vi "initialise.vi"(8 "error in (no error)":errorcluster, 11 "DL090211FrameImageAssembler in":refnum<class "ImageAssemblerDL090211Frame.lvclass">) -> (0 "error out":errorcluster, 3 "DL090211FrameImageAssembler out":refnum<class "ImageAssemblerDL090211Frame.lvclass">)   [LabVIEW 2010, in "ImageAssemblerDL090211Frame.lvclass"]
doc: "The dynamic dispatch-version of this VI initalises the plug-in object by allocating and initalising any dynamic resources need."
uses:
  ImageAssemblerDL090211Frame.lvclass
  ImageAssemblerDL090211Scaffold/ImageAssemblerDL090211Scaffold/ImageAssemblerDL090211Scaffold.lvclass
  common/arrays/pixel_raw_data_array.ctl
  ImageAssemblerDL090211Frame.lvclass/ImageAssemblerDL090211Frame.ctl
  common/classes/Image/Image/Image.lvclass
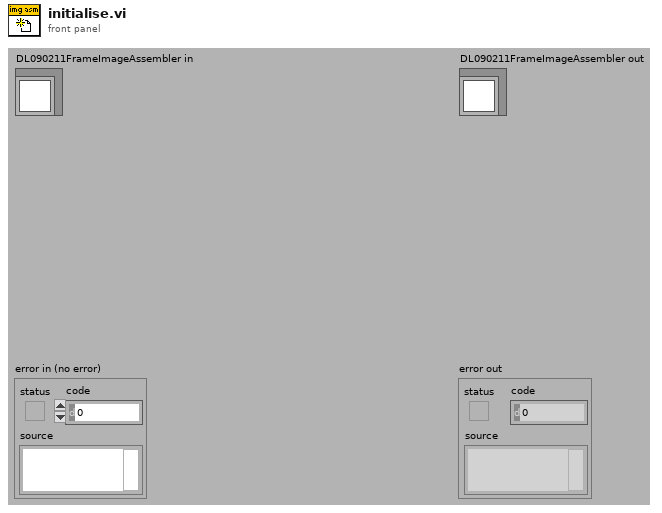
[diagram p1: front panel]
types:
  T1 = typedef "pixel_raw_data_array.ctl" = dbl[][]
  T2 = typedef "Image Type" = u32
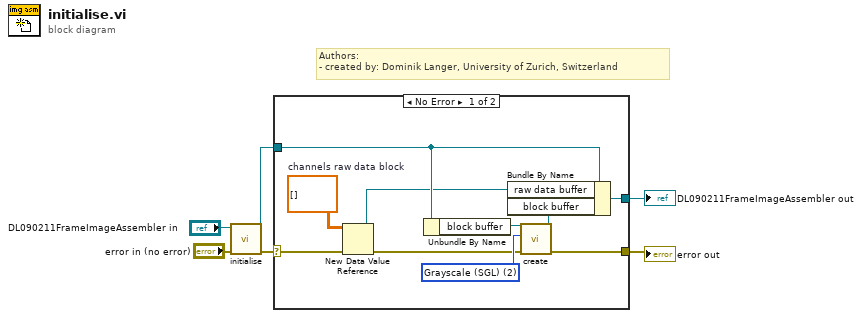
[diagram p0: block diagram]
diagram:
  # "Authors: \n- created by: Dominik Langer, University of Zurich, Switzerland"
  n1 = call-parent "initialise.vi"("error in (no error)"="error in (no error)", "GenericPlugin in"="DL090211FrameImageAssembler in") -> ("error out"=w4:errorcluster, "GenericPlugin out"=w3:refnum<class "ImageAssemblerDL090211Frame.lvclass">)  [unwired: 8 out]
  n2 = case shown="No Error" w4 {
    selector: w4 -> [w12 w17]
    tunnel: w3 -> [w13 w18]
    tunnel: [w8 w17] -> w2
    tunnel: [w7 w18] -> w1
    frame No Error {
      w11 = T1 []  # channels raw data block
      w16 = T2 2 items=["Grayscale (U8)", "Grayscale (I16)", "Grayscale (SGL)", "Complex (CSG)", "RGB (U32)", "HSL (U32)", "RGB (U64)", "Grayscale (U16)"] ("Image Type")
      n3 = New Data Value Reference(data value=w11, error in=w12) -> (data value reference=w9:refnum<data-value>, error out=w10:errorcluster)
      n4 = Unbundle By Name(w13) -> ("block buffer"=w15:refnum<class "Image.lvclass">)
      n5 = call "create.vi"("error in (no error)"=w10, "Image Type"=w16, "Image in"=w15) -> ("error out"=w8:errorcluster, "Image out"=w14:refnum<class "Image.lvclass">)  [unwired: 1 in, 6 out]
      n6 = Bundle By Name(cluster=w13, "raw data buffer"=w9, "block buffer"=w14) -> (w7:refnum<class "ImageAssemblerDL090211Frame.lvclass">)
    }
    frame Error {
    }
  }
  "error out" <- w2
  "DL090211FrameImageAssembler out" <- w1
